vi "OCT.vi"() -> ()   [LabVIEW 2014]
doc: "I. Description:\nThis example demonstrates how to acquire a continuous amount of data (Waveform) using the DAQ device's internal clock.\n\nII. Instructions for Running:\n1. Create an analog input voltage channel.\n2. Set the rate for the sample clock. Additionally, define the sample mode to be continuous.\n3. Call the Start VI to start the acquisition.\n4. Read the waveform data in a loop until the user hits the stop button or an error occurs.\nNote: This example reads data from one or more channels and returns an array of data. Use the Index Array function to access an individual channel of data.\n5. Call the Clear Task VI to clear the Task.\n6. Use the popup dialog box to display an error if any.\n\nIV. I/O Connections Overview:\nMake sure your signal input terminal matches the Physical Channel I/O Control. For further connection information, refer to your hardware reference manual."
uses:
  ATS-VI/ATS_ctl/Device_Ctrl.ctl
  ATS-VI/ATS_ctl/ATS_Async_Ctrl.ctl
  ATS-VI/ATS_ctl/ATS_Async_Mode.ctl
  ATS-VI/ATS_ctl/ATS_DMA_Channel.ctl
  ATS-VI/ATS_ctl/ATS_ReadSamples.ctl
  ATS-VI/ATS_ctl/ATS_Check_Ctrl.ctl
  ATS-VI/ATS_ctl/ClockSource.ctl
  Galvo VIs/galvo_states.ctl
  Signal Processing/processing_states.ctl
  En Face/En Face States.ctl
  Saving Data/Saving Data States.ctl
  Type Defs/OCT Hardware States.ctl
  ATS-VI/ATS_ctl/Range.ctl
  ATS-VI/ATS_ctl/Impedance.ctl
  Type Defs/OCT Imaging Parameters Cluster.ctl
  Signal Processing/Display Raw Data states.ctl
  ATS-VI/ATS_ctl/Record.ctl
  ATS-VI/ATS_ctl/ClockRate.ctl
  ATS-VI/ATS_ctl/ClockEdge.ctl
  ATS-VI/ATS_ctl/Clock.ctl
  ATS-VI/ATS_ctl/Coupling.ctl
  ATS-VI/ATS_ctl/Bandwidth.ctl
  ATS-VI/ATS_ctl/InputCtrl.ctl
  ATS-VI/ATS_ctl/TriggerOperation.ctl
  ATS-VI/ATS_ctl/TriggerEngine.ctl
  ATS-VI/ATS_ctl/ExtTrigRange.ctl
  ATS-VI/ATS_ctl/ExtTrigger.ctl
  ATS-VI/ATS_ctl/Trigger.ctl
  ATS-VI/ATS_ctl/ATS_Global.ctl
  En Face/En Face Depth Parameters.ctl
  DAQ Status States.ctl
  Classes/DAQ/ATS9462/ATS9462 Class.lvclass
  Type Defs/Display States.ctl
  ATS-VI/ATS_ctl/ATS_Async_Setting.ctl
  Type Defs/OCT DAQ Channel Data Type.ctl
panel:
  out "Background Array":u16[](array[numeric])
  in  "Calibrate":bool
  in  "Save Sweep Button":bool
  in  "Linear?":bool
  in  "Data Format":T1
  out "BScan":sgl[][](graph)
  in  "Display":T2
  in  "Save Sweep":bool
  in  "Stop Button":bool
  out "B-Scans Per Buffer":i32=1
  out "Current State":T3=enum."Aquire and Save"
  in  "Channels":tag="Dev2/ao0:1"
  in  "Trigger Source":tag="/Dev2/PFI7"
  in  "Imaging Parameters":T4={"Points Per A-Scan"=0, "A-Scans per B-Scan"=0, "Voltage Range"=1.0, "Card Resolution (bits)"=12}
  out "First Time?":bool=TRUE
  out "Save Data":bool
  in  "Async_Setting":T5
  out "Processing Finished":bool
  in  "OCT Hardware States":T6=enum."Acquire Clock"
  out "Save State":T7=enum."Do Nothing"
  out "Clock Length":u32=9184
  out "Reset DAQ":bool
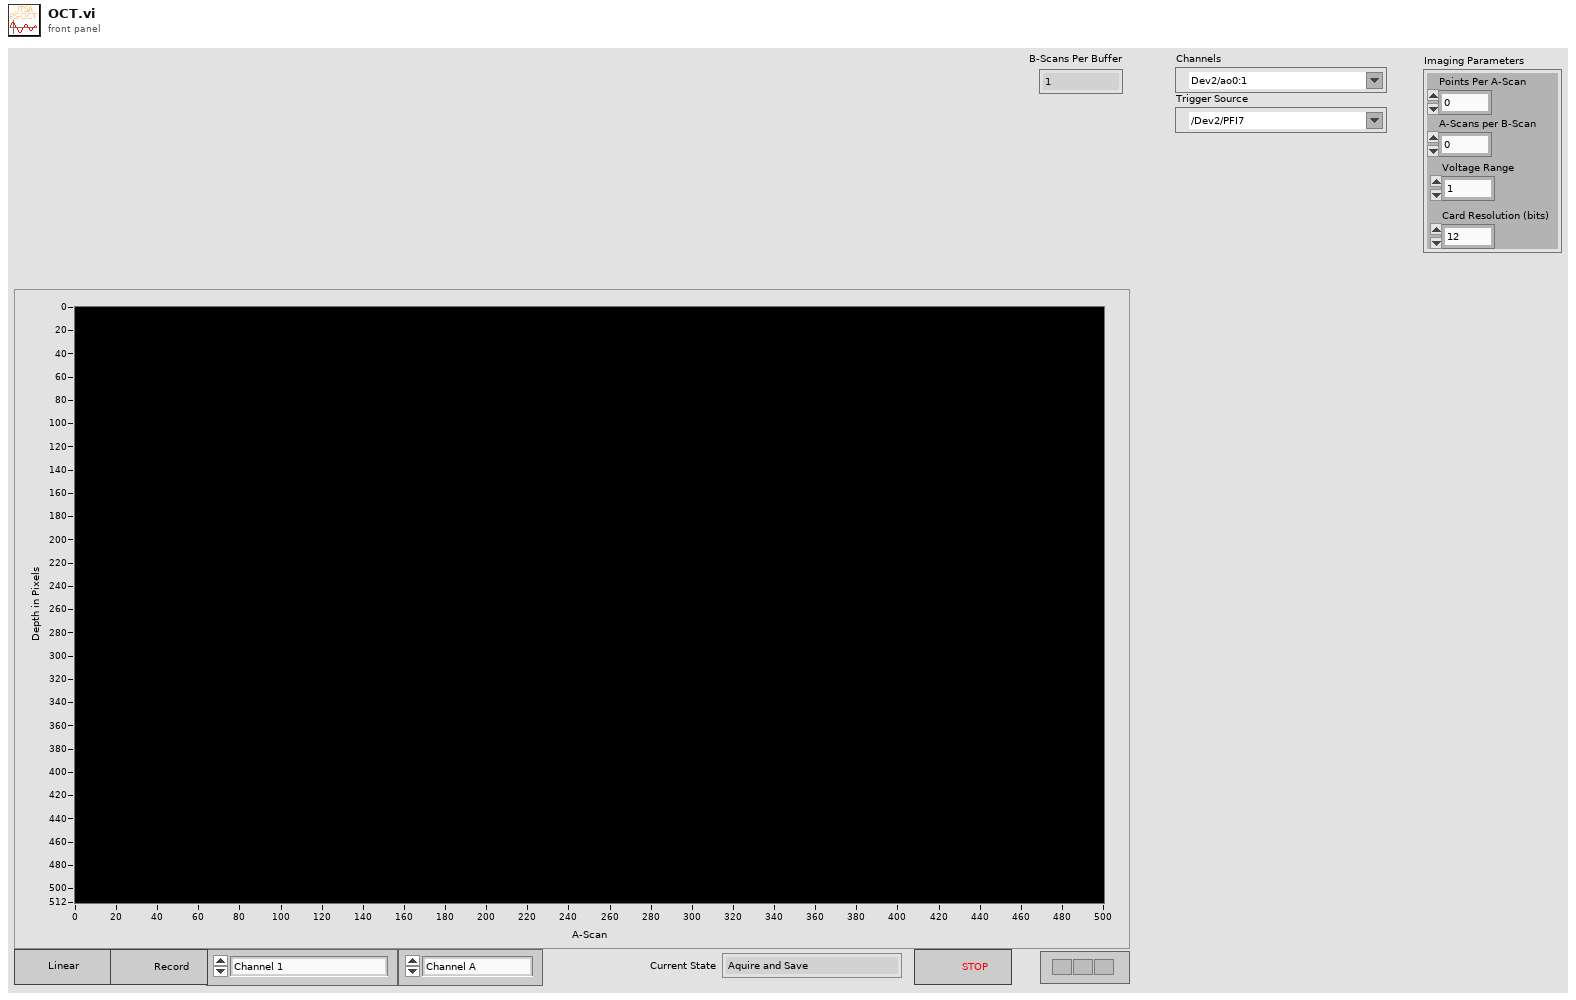
[diagram p1: front panel]
types:
  T1 = typedef "OCT DAQ Channel Data Type.ctl" = enum16{"Channel 1", "Channel 2", "Channel 1 and 2"}
  T2 = typedef "Display States.ctl" = enum16{"Channel A", "Channel B"}
  T3 = typedef "OCT Hardware States.ctl" = enum16{"Acquire Data", "Aquire and Save", "Reset DAQ", "Background Subtraction", "Acquire Background", "Update DAQ Parameters", "Stop", "Set Clock", "Initialize DAQ", "Set Resampling Array"}
  T4 = typedef "OCT Imaging Parameters Cluster.ctl" = cluster{"Points Per A-Scan":i32, "A-Scans per B-Scan":i32, "Voltage Range":sgl, "Card Resolution (bits)":u16}
  T5 = typedef "ATS_Async_Setting.ctl" = cluster{"UseHeader":u32, "Rec/Buffer":u32, "Total_Rec":u32, "DataBuffer":bool, "GetProcessedData":bool}
  T6 = typedef "OCT Hardware States.ctl" = enum16{"Acquire Data", "Aquire and Save", "Allocate OpenCL Memory", "Delete OpenCL Memory", "Background Subtraction", "Acquire Background", "K-Space Calibration", "Update DAQ Parameters", "Initialize Clock", "Stop", "Wait", "Acquire Clock", "Initialize DAQ", "Set Resampling Array"}
  T7 = typedef "Saving Data States.ctl" = enum16{"Get Queue Size", "Get Queue", "Get Timeout", "Flush Queue", "Close Files", "Create Files", "Do Nothing", "Initialize", "Enqueue Data", "Save Data", "Shutdown"}
  T8 = typedef "ATS_Global.ctl" = cluster{"Record":T9, "Clock":T10, "Input A":T14, "Input B":T14, "Trigger":T19}
  T9 = typedef "Record.ctl" = cluster{"Count":u32, "Presize":u32, "Length":u32}
  T10 = typedef "Clock.ctl" = cluster{"ClckSource":T11, "ClckRate":T12, "ClckEdge":T13, "Decimation":u32}
  T11 = typedef "ClockSource.ctl" = enum16{"Internal", "External", "Medium Ext.", "Slow Ext.", "Ext. AC", "Ext. DC", "Ext. (PLL)"}
  T12 = typedef "ClockRate.ctl" = u32
  T13 = typedef "ClockEdge.ctl" = u16
  T14 = typedef "InputCtrl.ctl" = cluster{"Coupling":T15, "Range":T16, "Impedance":T17, "Bandwidth":T18}
  T15 = typedef "Coupling.ctl" = enum16{"AC", "DC"}
  T16 = typedef "Range.ctl" = u32
  T17 = typedef "Impedance.ctl" = enum16{"1M ohms", "50 ohms"}
  T18 = typedef "Bandwidth.ctl" = enum16{"Full Bandwidth", "Reduce Bandwidth"}
  T19 = typedef "Trigger.ctl" = cluster{"TrigOperation":T20, "Timeout (s)":dbl, "Trig. Delay":u32, "Engine X":T21, "Engine Y":T21, "ExtTrigControl":T22}
  T20 = typedef "TriggerOperation.ctl" = enum16{"Only X", "Only Y", "X or Y", "X and Y", "X xor Y", "X and not Y", "not X and Y"}
  T21 = typedef "TriggerEngine.ctl" = cluster{"Source":enum32{"Chan_A", "Chan_B", "External", "Disable"}, "Slope":enum32{"Positive", "Negative"}, "Level":u32}
  T22 = typedef "ExtTrigger.ctl" = cluster{"Coupling":T15, "Range":T23}
  T23 = typedef "ExtTrigRange.ctl" = enum16{"1 V", "5 V", "TTL"}
  T24 = typedef "galvo_states.ctl" = enum16{"Reset", "Reset Galvos?", "Center Galvos", "Register Callback", "Get Scan Parameters", "Show", "Initialize", "Run Raster", "Load Raster", "Run Circle", "Shutdown"}
  T25 = typedef "OCT Hardware States.ctl" = enum16{"Acquire Data", "Initialize Laser", "Initialize Galvos", "Startup", "Reset DAQ", "Background Subtraction", "Acquire Background", "Update DAQ Parameters", "Stop", "Set Clock", "Initialize DAQ", "Set Resampling Array", "Save Sweep", "Configure Laser"}
  T26 = typedef "En Face Depth Parameters.ctl" = cluster{"En Face Start\nDepth":i32, "En Face End\nDepth":i32}
  T27 = typedef "processing_states.ctl" = enum16{"Initialize", "Set Background", "Update Imaging Parameters", "Get Queue", "Process Data", "Get Size", "Flush Data", "Set Reample Array", "Get Last Processed BScan", "Shutdown"}
  T28 = typedef "En Face States.ctl" = enum16{"Save BMP", "Show", "Clear En Face", "Update EnFace"}
  T29 = typedef "Galvo.lvclass/Scanning Cluster.ctl" = cluster{"Fast Axis Offset":sgl, "Slow Axis Offset":sgl, "Slow Axis Amp":sgl, "Fast Axis Amp":sgl, "Scan Pattern":enum16{"Raster"}}
  T30 = typedef "Processed OCT Data.ctl" = cluster{"Intensity A":sgl[][][], "Intensity B":sgl[][][]}
  T31 = typedef "ATS_Async_Ctrl.ctl" = enum16{"SetupDMA", "StartCapture", "Get", "Get_Stream", "Abort", "Stop"}
  T32 = typedef "ATS_ReadSamples.ctl" = cluster{"Offset":i32, "Length":u32}
  T33 = typedef "ATS_DMA_Channel.ctl" = enum16{"Channel_A", "Channel_B", "A & B"}
  T34 = typedef "ATS_Async_Mode.ctl" = enum16{"Continuous", "Triggered", "No-Pre-Trigger", "Traditional"}
  T35 = typedef "ATS_Check_Ctrl.ctl" = enum16{"None", "NO_ATS9462", "ATS9462_Traditional", "Verify Board", "OnBoard Memory", "Board & Memory", "Master/Slave", "NO Master/Slave"}
  T36 = typedef "Device_Ctrl.ctl" = enum16{"Status", "About", "Arm", "ForceTrig", "Abort", "Initialize", "Init (NoPreset)", "Info", "Close", "Calibrate", "SetManually", "LED_ON", "LED_OFF"}
  T37 = typedef "DAQ Status States.ctl" = enum16{"Get", "Show"}
  T38 = typedef "ATS_Async_Status.ctl" = cluster{"Start DMA":bool, "StartCapture":bool, "Valid":bool, "Completed":bool, "InProgress":bool, "Timeout":bool, "Overflow":bool, "Error":bool}
  T39 = typedef "Display Raw Data states.ctl" = enum16{"Add Raw", "Add Processed", "Show"}
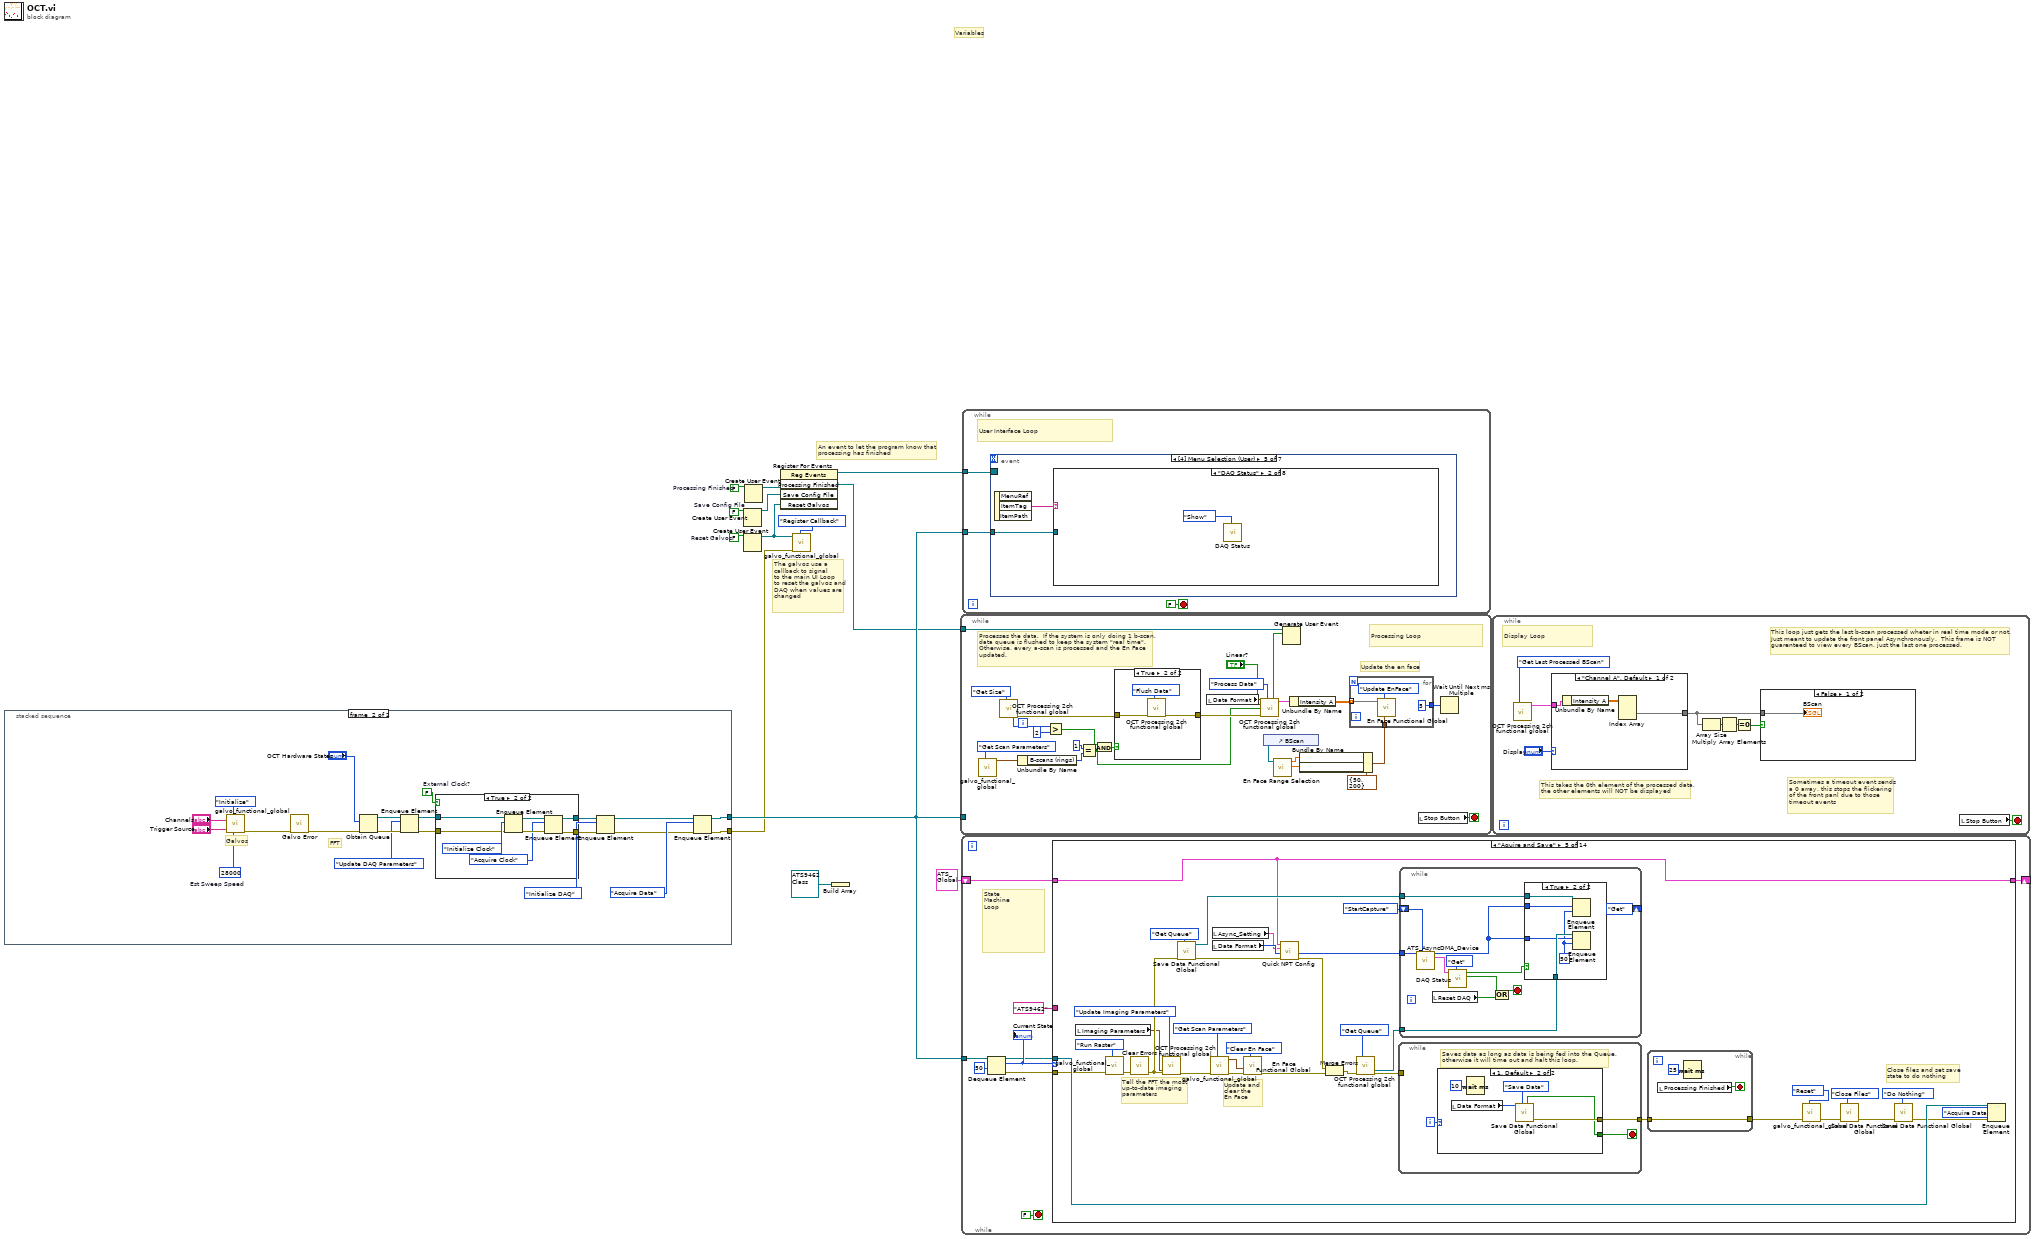
[diagram p0: block diagram]
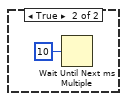
[diagram p3: hidden frame]
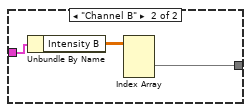
[diagram p4: hidden frame]
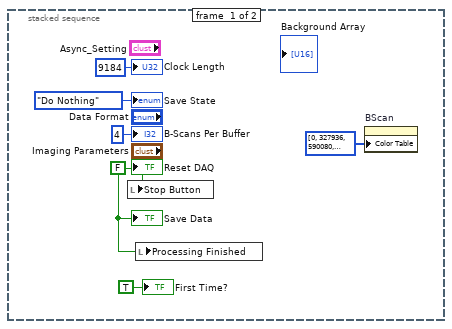
[diagram p5: hidden frame]
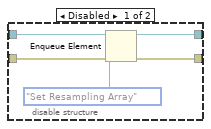
[diagram p7: hidden frame]
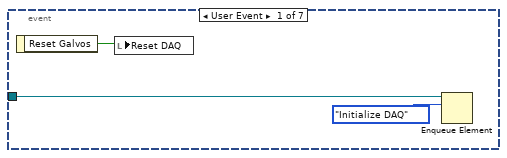
[diagram p8: hidden frame]
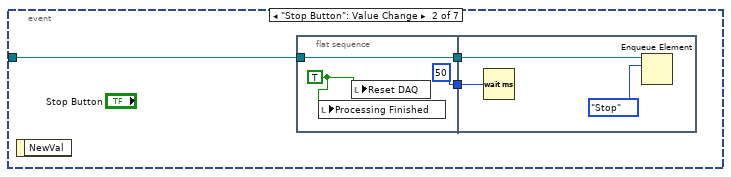
[diagram p9: hidden frame]
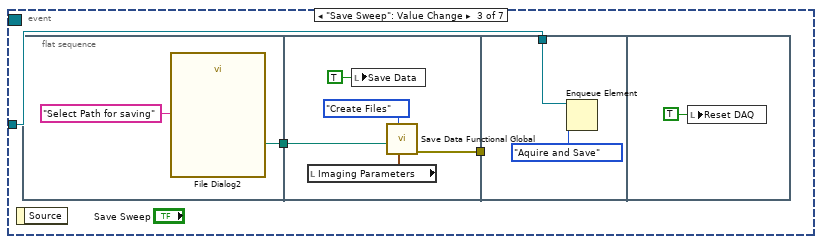
[diagram p10: hidden frame]
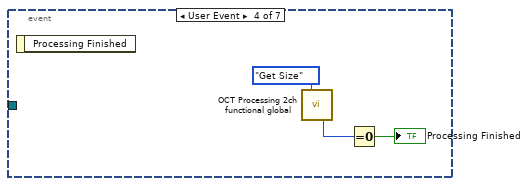
[diagram p11: hidden frame]
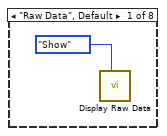
[diagram p12: hidden frame]
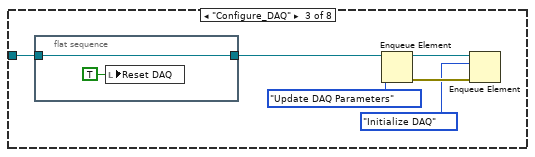
[diagram p13: hidden frame]
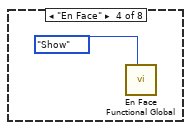
[diagram p14: hidden frame]
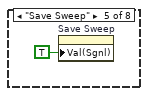
[diagram p15: hidden frame]
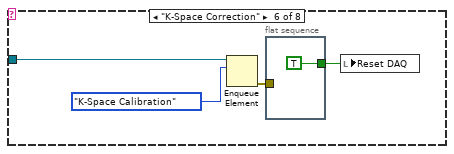
[diagram p16: hidden frame]
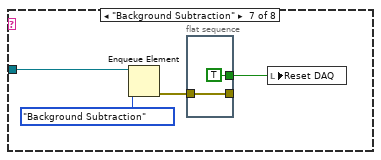
[diagram p17: hidden frame]
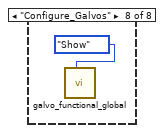
[diagram p18: hidden frame]
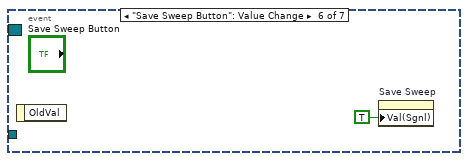
[diagram p19: hidden frame]
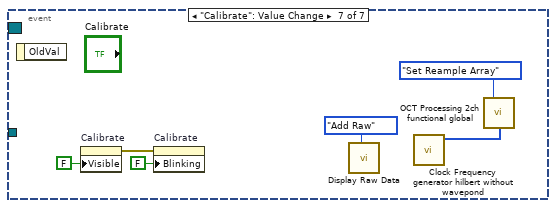
[diagram p20: hidden frame]
diagram:
  w7 = FALSE  # Reset Galvos
  w10 = FALSE  # Save Config File
  w13 = FALSE  # Processing Finished
  # "The galvos use a \ncallback to signal\nto the main UI Loop\nto reset the galvos and\nDAQ when values are\nchanged"
  # "An event to let the program know that\nprocessing has finished"
  # "Variables"
  n1 = stacked-sequence {
    tunnel: [_ w28] -> w11
    tunnel: [_ w27] -> w3
    frame #0 {
      w16 = FALSE ("Sweep Ready for saving")
      n2 = local write "Stop Button"(w16) -> ()
      n3 = local write "Processing Finished"(w16) -> ()
      n4 = property on="BScan" class="IntGraph (strict)"("Color Table"=u32[] [0, 327936, 590080, 852224, 983296, 1114624, 1180160, 1311232, 1442304, 1573632, 1704704, 1770240, 1901312, 1966848, 2098176, 2163712, 2294784, 2491392, 2557184, 2688256, 2753792, 2884864, 2950656, 3081728, 3147264, 3344129, 3475457, 3540993, 3672321, 3738113, 3869185, 3934977, 4066305, 4197633, 4328961, 4394497, 4460289, 4591617, 4657409, 4788481, 4854273, 4985601, 5116929, 5248257, 5314049, 5379841, 5511169, 5576961, 5708033, 5773825, 5905153, 6036482, 6167810, 6233346, 6299138, 6430466, 6496258, 6562050, 6693634, 6759426, 6890754, 7022082, 7087874, 7153666, 7284994, 7350786, 7482114, 7547906, 7613698, 7745026, 7876354, 8007682, 8073474, 8139522, 8205314, 8336642, 8467970, 8533763, 8599555, 8665347, 8731139, 8862467, 8993795, 9059587, 9125380, 9191428, 9257220, 9388548, 9454340, 9520132, 9585924, 9717253, 9848837, 9914629, 9980165, 10045957, 10177541, 10243334, 10309126, 10375174, 10440966, 10572294, 10703623, 10769416, 10835208, 10901256, 10967049, 11033097, 11033609, 11099401, 11165450, 11231242, 11231754, 11297547, 11363339, 11429131, 11495180, 11495692, 11561740, 11693069, 11758861, 11759373, 11825165, 11891214, 11957006, 12022799, 12023311, 12089103, 12220944, 12286736, 12286736, 12352529, 12418577, 12484370, 12550162, 12615954, 12681747, 12747796, 12813588, 12813845, 12879894, 12945686, 13077015, 13142808, 13143064, 13208856, 13274905, 13340697, 13340953, 13472282, 13538075, 13604379, 13670172, 13735964, 13801757, 13867550, 13933343, 13999392, 13999648, 14065441, 14131234, 14197027, 14197541, 14263334, 14329383, 14395176, 14460969, 14592553, 14658346, 14724139, 14789932, 14790189, 14856238, 14922287, 14988080, 15053873, 15054130, 15119923, 15185972, 15251765, 15317559, 15383353, 15449146, 15449660, 15515454, 15515968, 15516226, 15582021, 15582278, 15582536, 15648587, 15648844, 15714639, 15714897, 15715155, 15780949, 15781463, 15847256, 15847770, 15848028, 15913823, 15914081, 15979875, 15980133, 15980391, 16046441, 16046444, 16046703, 16046705, 16112500, 16113015, 16113274, 16113277, 16179072, 16179330, 16179588, 16245384, 16245387, 16245389, 16245648, 16311443, 16376982, 16377241, 16377499, 16443294, 16443553, 16443555, 16443815, 16509866, 16510124, 16510127, 16575923, 16575924, 16576182, 16576441, 16576443, 16576702, 16576705, 16576963, 16577222, 16577224, 16577482, 16577485, 16577743, 16577745, 16578004, 16578262, 16578264, 16578523, 16578782, 16579040, 16579299, 16579301, 16579303, 16579562, 16579821]) -> ()  [unwired: 2 in, 2 out]
      "B-Scans Per Buffer" <- 4 ("B-Scans Per Buffer")
      "Clock Length" <- u32 9184 ("Clock Length")
      "Save State" <- Saving_Data_States."Do Nothing" ("Save State")
      "Reset DAQ" <- w16
      "Save Data" <- w16
      "First Time?" <- TRUE ("First Time?")
    }
    frame #1 {
      w32 = 28000  # Est Sweep Speed
      w33 = FALSE  # External Clock?
      # "FFT"
      # "Galvos"
      n5 = call "galvo_functional_global.vi"("Est Sweep Speed"=w32, "State"=galvo_states."Initialize", "Trigger Source"="Trigger Source", "Analog Output"="Channels") -> ("error out"=w21:errorcluster)  [unwired: 6 in, 1 out]
      n6 = call "Galvo Error.vi"("error in (no error)"=w21) -> ("error out"=w20:errorcluster)  [unwired: 10 in]
      n7 = Obtain Queue(element data type="OCT Hardware States", error in (no error)=w20) -> (queue out=w30:refnum<queue>, error out=w31:errorcluster)  [unwired: 3 in, 1 out]
      n8 = Enqueue Element(queue=w30, element=OCT_Hardware_States."Update DAQ Parameters", error in (no error)=w31) -> (queue out=w25:refnum<queue>, error out=w24:errorcluster)  [unwired: 1 in, 1 out]
      n9 = case shown="True" w33 {
        tunnel: [w41 w57] -> w40
        tunnel: [w42 w56] -> w39
        tunnel: w25 -> [w44 w53]
        tunnel: w24 -> [w43 w52]
        frame False {
          n10 = disable-structure shown="Enabled" {
            disable-tunnel: w44 -> [w49 w51]
            disable-tunnel: w43 -> [w48 w50]
            disable-tunnel: [w47 w50] -> w42
            disable-tunnel: [w46 w51] -> w41
            frame Disabled {
              n11 = Enqueue Element(queue=w49, element=OCT_Hardware_States."Set Resampling Array", error in (no error)=w48) -> (queue out=w46:refnum<queue>, error out=w47:errorcluster)  [unwired: 1 in, 1 out]
            }
            frame Enabled {
            }
          }
        }
        frame True {
          n12 = Enqueue Element(queue=w53, element=OCT_Hardware_States."Initialize Clock", error in (no error)=w52) -> (queue out=w59:refnum<queue>, error out=w58:errorcluster)  [unwired: 1 in, 1 out]
          n13 = Enqueue Element(queue=w59, element=OCT_Hardware_States."Acquire Clock", error in (no error)=w58) -> (queue out=w57:refnum<queue>, error out=w56:errorcluster)  [unwired: 1 in, 1 out]
        }
      }
      n14 = Enqueue Element(queue=w40, element=OCT_Hardware_States."Initialize DAQ", error in (no error)=w39) -> (queue out=w22:refnum<queue>, error out=w23:errorcluster)  [unwired: 1 in, 1 out]
      n15 = Enqueue Element(queue=w22, element=OCT_Hardware_States."Acquire Data", error in (no error)=w23) -> (queue out=w28:refnum<queue>, error out=w27:errorcluster)  [unwired: 1 in, 1 out]
    }
  }
  n16 = Create User Event(user event datatype=w10) -> (user event=w9:refnum<user-event>)  [unwired: 1 in, 1 out]
  n17 = Create User Event(user event datatype=w7) -> (user event=w6:refnum<user-event>)  [unwired: 1 in, 1 out]
  n18 = Create User Event(user event datatype=w13) -> (user event=w8:refnum<user-event>)  [unwired: 1 in, 1 out]
  n19 = register-events(w8, w9, w6) -> (reference out=w12:refnum<event-registration>)  [unwired: 2 in, 1 out]
  n20 = call "galvo_functional_global.vi"("State"=galvo_states."Register Callback", "error in (no error)"=w3, "user event out"=w6) -> ()  [unwired: 7 in, 2 out]
  n21 = Build Array(refnum<class "ATS9462 Class.lvclass"> refnum ("ATS9462 Class.lvclass")) -> (w1:refnum<class "ATS9462 Class.lvclass">[])
  n22 = while {
    tunnel: w8 -> [w75]
    tunnel: w11 -> [_]
    stop <- w85 stop-if-true
    # "Processing Loop"
    # "Update the en face"
    # "Processes the data.  If the system is only doing 1 b-scan, \ndata queue is flushed to keep the system \"real time\".\nOtherwise, every a-scan is processed and the En Face\nupdated."
    n23 = call "galvo_functional_global.vi"("State"=galvo_states."Get Scan Parameters") -> ("Scanning Output"=w69:T29)  [unwired: 9 in, 1 out]
    n24 = call "OCT Processing 2ch functional global.vi"("State"=processing_states."Get Size") -> ("# elements in queue"=w81:i32, "error out"=w72:errorcluster)  [unwired: 10 in, 3 out]
    n25 = Unbundle By Name(w69) -> ("B-scans (rings)"=w77:u32)
    n26 = Greater?(x=w81, y=2) -> (0:w82:bool)
    n27 = Equal?(x=u32 1, y=w77) -> (x = y?=w65:bool)
    n28 = And(x=w82, y=w65) -> (x .and. y?=w70:bool)
    n29 = case shown="True" w70 {
      tunnel: w72 -> [w90 w93]
      tunnel: [w90 w92] -> w71
      frame False {
      }
      frame True {
        n30 = call "OCT Processing 2ch functional global.vi"("State"=processing_states."Flush Data", "error in (no error)"=w93) -> ("error out"=w92:errorcluster)  [unwired: 9 in, 4 out]
      }
    }
    n31 = local read "Data Format"() -> (w76:T1)
    n32 = call "OCT Processing 2ch functional global.vi"("Data Format"=w76, "State"=processing_states."Process Data", "Linear?"="Linear?", "Real Time"=w65, "error in (no error)"=w71) -> ("Time Out"=w74:bool, "Processed OCT Data"=w79:T30)  [unwired: 6 in, 3 out]
    n33 = control-ref of="BScan"() -> (w64:refnum<vi>)
    n34 = call "En Face Range Selection.vi"("IntensityGraph in"=w64) -> ("Lower En Face"=w61:dbl, "Upper En Face"=w62:dbl)  [unwired: 9 in]
    n35 = Generate User Event(user event=w75, event data cluster=w74) -> ()  [unwired: 2 in, 2 out]
    n36 = Unbundle By Name(w79) -> ("Intensity A"=w73:sgl[][][])
    n37 = Bundle By Name(cluster=T26 {"En Face Start\nDepth"=50, "En Face End\nDepth"=200} ("En Face Parameters"), "En Face Start\nDepth"=w62, "En Face End\nDepth"=w61) -> (w60:T26)
    n38 = for {
      tunnel: w73 -> [w88] mode=indexing
      tunnel: [u32 5 ("millisecond multiple")] -> w67
      tunnel: w60 -> [w86]
      n39 = call "En Face Functional Global.vi"(6:w86, 7:En_Face_States."Update EnFace" ("En Face States"), "Intensity Graph 2"=w88) -> ()  [unwired: 7 in, 2 out]
    }
    n40 = local read "Stop Button"() -> (w85:bool)
    n41 = Wait Until Next ms Multiple(millisecond multiple=w67) -> ()  [unwired: 1 out]
  }
  n42 = while {
    tunnel: w11 -> [w102]
    shift-right: [w96] -> _
    shift-left: T8 {"Record"={"Count"=0, "Presize"=0, "Length"=0}, "Clock"={"ClckSource"=enum."Internal", "ClckRate"=0, "ClckEdge"=0, "Decimation"=0}, "Input A"={"Coupling"=enum."DC", "Range"=12, "Impedance"=enum."1M ohms", "Bandwidth"=enum."Full Bandwidth"}, "Input B"={"Coupling"=enum."DC", "Range"=12, "Impedance"=enum."1M ohms", "Bandwidth"=enum."Full Bandwidth"}, "Trigger"={"TrigOperation"=enum."Only X", "Timeout (s)"=-1.0, "Trig. Delay"=0, "Engine X"={"Source"=enum."Chan_A", "Slope"=enum."Positive", "Level"=0}, "Engine Y"={"Source"=enum."Chan_A", "Slope"=enum."Positive", "Level"=0}, "ExtTrigControl"={"Coupling"=enum."AC", "Range"=enum."1 V"}}} ("Value") -> [w95]
    stop <- FALSE stop-if-true
    # "State\nMachine\nLoop"
    n43 = Dequeue Element(queue=w102, timeout in ms (-1)=50) -> (queue out=w98:refnum<queue>, element=w100:T6, error out=w99:errorcluster)  [unwired: 1 in, 1 out]
    "Current State" <- w100
    n44 = case shown="\"Aquire and Save\"" w100 {
      tunnel: w99 -> [_ w146 w203 w255 w309 _ w367 _ _ _ w405 w413 _ _]
      tunnel: w98 -> [_ _ w204 w254 w323 _ w368 _ _ _ w406 w411 _ _]
      tunnel: "ATS9462" ("BoardToVerify") -> [_ w160 _ _ _ _ _ w375 _ _ _ _ _ _]
      tunnel: [w119 w154 w220 w266 w298 w357 w359 w374 w390 w391 w401 w415 w418 w419] -> w96
      tunnel: w95 -> [w119 w153 w220 w266 w298 w357 w359 w374 w390 _ w401 w415 w418 w419]
      frame "Acquire Clock" {
        w106 = 0 ("DeviceIn")
        n45 = local read "Clock Length"() -> (w108:u32)
        n46 = local read "Async_Setting"() -> (w104:T5)
        n47 = Bundle By Name(cluster=w104, "UseHeader"=u32 0, "Rec/Buffer"=u32 125, "Total_Rec"=u32 0) -> (w105:T5)
        n48 = Unbundle By Name(w119) -> ("Record.Presize"=w109:u32)
        n49 = Bundle By Name(cluster=T32 {"Offset"=0, "Length"=0} ("ReadSamples"), "Length"=w108, "Offset"=w109) -> (w107:T32)
        n50 = call "ATS_AsyncDMA_Device.vi"("DeviceIn"=w106, "ATS_Async_Ctrl"=ATS_Async_Ctrl."SetupDMA" ("ATS_DMA_Ctrl"), "Async_Mode"=ATS_Async_Mode."Traditional", "Async_Setting"=w105, "Channel"=ATS_DMA_Channel."Channel_B", "ReadSamples"=w107, "Start Now / Wait"=TRUE) -> ("Buffer"=w114:u16[])  [unwired: 4 in, 4 out]
        n51 = while {
          tunnel: w114 -> [_]
          shift-right: [ATS_Async_Ctrl."Get" ("ATS_Async_Ctrl")] -> _
          shift-left: ATS_Async_Ctrl."StartCapture" ("ATS_Async_Ctrl") -> [w128]
          tunnel: w106 -> [w123]
          stop <- w126 stop-if-true
          n52 = call "ATS_AsyncDMA_Device.vi"("DeviceIn"=w123, "ATS_Async_Ctrl"=w128) -> ("Buffer"=w121:u16[], "Async_Status"=w120:T38)  [unwired: 9 in, 3 out]
          n53 = Unbundle By Name(w120) -> ("Valid"=w122:bool, "Completed"=w130:bool, "Start DMA"=w131:bool, "Timeout"=w132:bool, "Error"=w129:bool)
          n54 = local read "Clock Length"() -> (w124:u32)
          n55 = Compound Arithmetic op=OR(w130, invert w131, w132, w129) -> (w125:bool)
          n56 = case shown="True" w122 {
            selector: w122 -> [w133 w136]
            tunnel: w121 -> [_ w135]
            tunnel: [w133 w136] -> w126
            tunnel: w125 -> [_ _]
            tunnel: w124 -> [_ w134]
            frame False {
            }
            frame True {
              n57 = Array Subset(array=w135, length=w134) -> (w137:u16[])  [unwired: 1 in]
              n58 = call "Clock Frequency generator hilbert.vi"(7:6300.0 ("Sweep Speed"), "Acquisition speed (S/s)"=180000000.0 ("Sweep Speed"), "k-space signal in"=w137, "number of frequency updates"=4385) -> ("Error Out"=w142:errorcluster, "frequency\nsteps"=w141:i32)  [unwired: 6 in]
              n59 = call "wavepond sequence.vi"("Error In"=w142, "Number of updates"=w141) -> ()  [unwired: 9 in, 1 out]
            }
          }
        }
      }
      frame "Initialize DAQ" {
        # "B-Scans per buffer should be around 4 if \ntaking more than 1 to minimize data transfer"
        # "If B Scans is 1, set total records to 0,\notherwise it should be A-Scans Per\nBScan times BScans"
        # "BScans Per Buffer"
        n60 = local read "First Time?"() -> (w157:bool)
        n61 = case shown="False" w157 {
          tunnel: [w186 w196] -> w182
          tunnel: w160 -> [_ w192]
          tunnel: [FALSE ("First Time?") FALSE ("First Time?")] -> w156
          frame False {
            n62 = flat-sequence {
              tunnel: [w188] -> w186
              frame #0 {
                w188 = 0 ("DeviceIn")
                n63 = call "ATS_AsyncDMA_Device.vi"("DeviceIn"=w188, "ATS_Async_Ctrl"=ATS_Async_Ctrl."Stop") -> ("ReadSamples_Out"=w191:T32)  [unwired: 9 in, 4 out]
                n64 = call "ATS_AsyncDMA_Device.vi"("DeviceIn"=w188, "ATS_Async_Ctrl"=ATS_Async_Ctrl."Abort", "ReadSamples"=w191) -> ()  [unwired: 8 in, 5 out]
              }
            }
          }
          frame True {
            n65 = call "ATS_Device.vi"("BoardToVerify"=w192, "ATS_Check"=ATS_Check_Ctrl."Verify Board", "DevCtrl"=Device_Ctrl."Initialize", "DeviceIn"=0 ("Device")) -> ("error out"=w194:errorcluster, "DeviceOut"=w198:i32)  [unwired: 1 in, 5 out]
            n66 = call "ATS_Device.vi"("error in (no error)"=w194, "DevCtrl"=Device_Ctrl."Abort", "DeviceIn"=w198) -> ("DeviceOut"=w196:i32)  [unwired: 2 in, 6 out]
          }
        }
        n67 = flat-sequence {
          tunnel: w146 -> [w184]
          tunnel: [w184] -> w147
          frame #0 {
            n68 = local write "Processing Finished"(FALSE ("Reset DAQ")) -> ()
            n69 = local write "Reset DAQ"(FALSE ("Reset DAQ")) -> ()
          }
        }
        n70 = call "Save Data Functional Global.vi"("States"=Saving_Data_States."Flush Queue", "error in (no error)"=w147) -> ("error out"=w149:errorcluster)  [unwired: 6 in, 3 out]
        n71 = call "OCT Processing 2ch functional global.vi"("State"=processing_states."Flush Data", "error in (no error)"=w149) -> ("error out"=w145:errorcluster)  [unwired: 9 in, 4 out]
        n72 = local write "First Time?"(w156) -> ()
        n73 = Unbundle By Name(w153) -> ("Record.Length"=w161:u32)
        n74 = call "ATS_MS_Set_Device.vi"("Set_Manually (F)"=FALSE, "Setup_In"=w153, "DeviceIn"=w182) -> ("Setup_Out"=w154:T8)  [unwired: 3 in, 5 out]
        n75 = call "galvo_functional_global.vi"("State"=galvo_states."Get Scan Parameters", "error in (no error)"=w145) -> ("Scanning Output"=w152:T29)  [unwired: 8 in, 1 out]
        n76 = Unbundle By Name(w152) -> ("B-scans (rings)"=w167:u32, "A(cluster)/B"=w177:u32, "B-scans (rings)"=w172:u32, "A(cluster)/B"=w171:u32, "B-scans (rings)"=w169:u32, "A(cluster)/B"=w163:u32)
        n77 = local read "Async_Setting"() -> (w159:T5)
        n78 = Not Equal?(x=w169, y=u32 1 ("x")) -> (x != y?=w170:bool)
        n79 = Equal?(x=u32 1, y=w167) -> (x = y?=w173:bool)
        n80 = local read "B-Scans Per Buffer"() -> (w155:i32)
        n81 = Select(t=u32 4 ("y"), s=w173, f=w155) -> (s? t:f=w175:u32)
        n82 = Multiply(x=w172, y=w171) -> (x*y=w166:u32)
        n83 = Select(t=w166, s=w170, f=u32 0 ("Total_Rec")) -> (s? t:f=w180:u32)
        n84 = Multiply(x=w175, y=w177) -> (x*y=w178:u32)
        n85 = Bundle By Name(cluster=T4 {"Points Per A-Scan"=0, "A-Scans per B-Scan"=0, "Voltage Range"=4.0, "Card Resolution (bits)"=16} ("Imaging Parameters"), "Points Per A-Scan"=w161, "A-Scans per B-Scan"=w163, "Voltage Range"=sgl 4.0, "Card Resolution (bits)"=u16 16) -> (w162:T4)
        n86 = Bundle By Name(cluster=w159, "UseHeader"=u32 0, "Rec/Buffer"=w178, "Total_Rec"=w180) -> (w158:T5)
        n87 = local write "Async_Setting"(w158) -> ()
        n88 = local write "Imaging Parameters"(w162) -> ()
      }
      frame "Acquire Data", Default {
        # "Update and \nclear the \nEn Face"
        # "Tell the FFT the most\nup-to-date imaging\nparameters"
        n89 = Enqueue Element(queue=w204, element=OCT_Hardware_States."Initialize DAQ", error in (no error)=w203) -> (error out=w201:errorcluster)  [unwired: 1 in, 2 out]
        n90 = local read "Imaging Parameters"() -> (w225:T4)
        n91 = call "galvo_functional_global.vi"("State"=galvo_states."Run Raster", "error in (no error)"=w201) -> ("error out"=w216:errorcluster)  [unwired: 8 in, 1 out]
        n92 = local read "Async_Setting"() -> (w224:T5)
        n93 = call <vilib>:"Clear Errors.vi"("error in (no error)"=w216) -> ("error out"=w215:errorcluster)  [unwired: 5 in, 1 out]
        n94 = call "OCT Processing 2ch functional global.vi"("State"=processing_states."Update Imaging Parameters", "Input Parameters"=w225, "error in (no error)"=w215) -> ("error out"=w208:errorcluster)  [unwired: 8 in, 4 out]
        n95 = local read "Data Format"() -> (w227:T1)
        n96 = call "galvo_functional_global.vi"("State"=galvo_states."Get Scan Parameters", "error in (no error)"=w208) -> ("error out"=w209:errorcluster, "Scanning Output"=w217:T29)  [unwired: 8 in]
        n97 = call "Quick NPT Config.vi"("error in (no error)"=w201, "Data Format"=w227, "Async_Setting"=w224, "Value"=w220) -> ("error out"=w205:errorcluster, "Device Out"=w230:i32, 3:w210)  [unwired: 4 in]
        n98 = call "En Face Functional Global.vi"(7:En_Face_States."Clear En Face" ("En Face States"), "Error In"=w209, 9:w217) -> ("Error Out"=w207:errorcluster)  [unwired: 7 in, 1 out]
        n99 = Merge Errors(w205, w207) -> (w206:errorcluster)
        n100 = call "OCT Processing 2ch functional global.vi"("State"=processing_states."Get Queue", "error in (no error)"=w206) -> ("queue out"=w222:refnum<queue>, "error out"=w214:errorcluster)  [unwired: 9 in, 3 out]
        n101 = while {
          tunnel: w230 -> [w250]
          shift-right: [ATS_Async_Ctrl."Get" ("ATS_Async_Ctrl")] -> _
          shift-left: ATS_Async_Ctrl."StartCapture" ("ATS_Async_Ctrl") -> [w249]
          tunnel: w222 -> [w245]
          tunnel: [w244] -> w221
          tunnel: w210 -> [w243]
          tunnel: w214 -> [w239]
          tunnel: [w239] -> w213
          stop <- w244 stop-if-true
          n102 = call "ATS_AsyncDMA_Device.vi"("DeviceIn"=w250, "ATS_Async_Ctrl"=w249) -> ("Buffer"=w247:u16[], "Async_Status"=w242:T38)  [unwired: 9 in, 3 out]
          n103 = local read "Reset DAQ"() -> (w246:bool)
          n104 = call "DAQ Status.vi"("Enum"=DAQ_Status_States."Get", "Async_Status"=w242) -> ("DAQ Error?"=w240:bool, "Valid"=w241:bool)  [unwired: 8 in]
          n105 = Compound Arithmetic op=OR(w240, w246) -> (w244:bool)
          n106 = case shown="True" w241 {
            tunnel: w247 -> [_ w251]
            tunnel: w245 -> [_ w253]
            tunnel: w243 -> [_ _]
            frame False {
              # "Do nothing"
            }
            frame True {
              n107 = Enqueue Element(queue=w253, element=w251, timeout in ms (-1)=50) -> ()  [unwired: 1 in, 3 out]
            }
          }
        }
        n108 = while {
          tunnel: w221 -> [w237]
          tunnel: [w234] -> w212
          tunnel: w213 -> [w234]
          stop <- w231 stop-if-true
          n109 = local read "Processing Finished"() -> (w236:bool)
          n110 = Wait (ms)(milliseconds to wait=u32 25) -> ()  [unwired: 1 out]
          n111 = local read "Reset DAQ"() -> (w232:bool)
          n112 = And(x=w237, y=w236) -> (x .and. y?=w233:bool)
          n113 = Or(x=w233, y=w232) -> (x .or. y?=w231:bool)
        }
        n114 = call "galvo_functional_global.vi"("State"=galvo_states."Reset", "error in (no error)"=w212) -> ()  [unwired: 8 in, 2 out]
      }
      frame "Acquire Background" {
        # "Update and \nclear the \nEn Face"
        # "Tell the FFT the most\nup-to-date imaging\nparameters"
        n115 = local read "Imaging Parameters"() -> (w268:T4)
        n116 = call "galvo_functional_global.vi"("State"=galvo_states."Run Raster", "error in (no error)"=w255) -> ("error out"=w263:errorcluster)  [unwired: 8 in, 1 out]
        n117 = local read "Async_Setting"() -> (w267:T5)
        n118 = call <vilib>:"Clear Errors.vi"("error in (no error)"=w263) -> ("error out"=w262:errorcluster)  [unwired: 5 in, 1 out]
        n119 = call "OCT Processing 2ch functional global.vi"("State"=processing_states."Update Imaging Parameters", "Input Parameters"=w268, "error in (no error)"=w262) -> ("error out"=w261:errorcluster)  [unwired: 8 in, 4 out]
        n120 = local read "Data Format"() -> (w269:T1)
        n121 = call "galvo_functional_global.vi"("State"=galvo_states."Get Scan Parameters", "error in (no error)"=w261) -> ("error out"=w259:errorcluster)  [unwired: 8 in, 1 out]
        n122 = call "Quick NPT Config.vi"("error in (no error)"=w255, "Data Format"=w269, "Async_Setting"=w267, "Value"=w266) -> ("error out"=w260:errorcluster, "Device Out"=w272:i32)  [unwired: 5 in]
        n123 = Merge Errors(w260, w259) -> (w256:errorcluster)
        n124 = while {
          tunnel: w272 -> [w282]
          shift-right: [ATS_Async_Ctrl."Get" ("ATS_Async_Ctrl")] -> _
          shift-left: ATS_Async_Ctrl."StartCapture" ("ATS_Async_Ctrl") -> [w281]
          tunnel: w256 -> [w278]
          tunnel: [w278] -> w257
          stop <- w274 stop-if-true
          n125 = local read "Imaging Parameters"() -> (w275:T4)
          n126 = call "ATS_AsyncDMA_Device.vi"("DeviceIn"=w282, "ATS_Async_Ctrl"=w281) -> ("Buffer"=w276:u16[], "Async_Status"=w279:T38)  [unwired: 9 in, 3 out]
          n127 = call "DAQ Status.vi"("Enum"=DAQ_Status_States."Get", "Async_Status"=w279) -> ("Valid"=w277:bool)  [unwired: 8 in, 1 out]
          n128 = case shown="True" w277 {
            selector: w277 -> [_ w287]
            tunnel: w276 -> [_ w291]
            tunnel: w275 -> [_ w290]
            tunnel: [FALSE w287] -> w274
            frame False {
            }
            frame True {
              n129 = Unbundle By Name(w290) -> ("A-Scans per B-Scan"=w289:i32, "Points Per A-Scan"=w288:i32)
              n130 = Reshape Array(w291, w289, w288) -> (w285:u16[][])
              n131 = call "Average BScan.vi"("B-Scan In"=w285) -> ("Averaged BScan"=w284:dbl[])  [unwired: 10 in]
              n132 = call "OCT Processing 2ch functional global.vi"("State"=processing_states."Set Background", "Background"=w284) -> ()  [unwired: 9 in, 5 out]
            }
          }
        }
        n133 = Enqueue Element(queue=w254, element=OCT_Hardware_States."Set Resampling Array", error in (no error)=w257) -> ()  [unwired: 1 in, 3 out]
      }
      frame "Aquire and Save" {
        # "Close files and set save \nstate to do nothing"
        # "Update and \nclear the \nEn Face"
        # "Tell the FFT the most\nup-to-date imaging\nparameters"
        n134 = local read "Imaging Parameters"() -> (w321:T4)
        n135 = call "galvo_functional_global.vi"("State"=galvo_states."Run Raster", "error in (no error)"=w309) -> ("error out"=w306:errorcluster)  [unwired: 8 in, 1 out]
        n136 = call <vilib>:"Clear Errors.vi"("error in (no error)"=w306) -> ("error out"=w326:errorcluster)  [unwired: 5 in, 1 out]
        n137 = call "OCT Processing 2ch functional global.vi"("State"=processing_states."Update Imaging Parameters", "Input Parameters"=w321, "error in (no error)"=w326) -> ("error out"=w295:errorcluster)  [unwired: 8 in, 4 out]
        n138 = call "Save Data Functional Global.vi"("States"=Saving_Data_States."Get Queue", "error in (no error)"=w326) -> ("error out"=w297:errorcluster, "Saving Queue Out"=w312:refnum<queue>)  [unwired: 6 in, 2 out]
        n139 = call "galvo_functional_global.vi"("State"=galvo_states."Get Scan Parameters", "error in (no error)"=w295) -> ("error out"=w296:errorcluster, "Scanning Output"=w307:T29)  [unwired: 8 in]
        n140 = local read "Async_Setting"() -> (w300:T5)
        n141 = local read "Data Format"() -> (w301:T1)
        n142 = call "En Face Functional Global.vi"(7:En_Face_States."Clear En Face" ("En Face States"), "Error In"=w296, 9:w307) -> ("Error Out"=w294:errorcluster)  [unwired: 7 in, 1 out]
        n143 = call "Quick NPT Config.vi"("error in (no error)"=w297, "Data Format"=w301, "Async_Setting"=w300, "Value"=w298) -> ("error out"=w293:errorcluster, "Device Out"=w299:i32)  [unwired: 5 in]
        n144 = Merge Errors(w293, w294) -> (w292:errorcluster)
        n145 = call "OCT Processing 2ch functional global.vi"("State"=processing_states."Get Queue", "error in (no error)"=w292) -> ("queue out"=w314:refnum<queue>, "error out"=w316:errorcluster)  [unwired: 9 in, 3 out]
        n146 = while {
          tunnel: w316 -> [_]
          tunnel: [w332] -> w303
          i -> [w331]
          stop <- w330 stop-if-true
          # "Saves data as long as data is being fed into the Queue,\notherwise it will time out and halt this loop."
          n147 = case shown="1, Default" w331 {
            tunnel: [FALSE w335] -> w330
            tunnel: [_ w336] -> w332
            frame 0 {
              # "Wait for data to Q up"
              n148 = Wait (ms)(milliseconds to wait=u32 500) -> ()  [unwired: 1 out]
            }
            frame 1, Default {
              n149 = local read "Data Format"() -> (w338:T1)
              n150 = Wait (ms)(milliseconds to wait=u32 10) -> ()  [unwired: 1 out]
              n151 = call "Save Data Functional Global.vi"("States"=Saving_Data_States."Save Data", "Data Format"=w338) -> ("error out"=w336:errorcluster, "Time Out"=w335:bool)  [unwired: 6 in, 2 out]
            }
          }
        }
        n152 = while {
          shift-right: [ATS_Async_Ctrl."Get" ("ATS_Async_Ctrl")] -> _
          shift-left: ATS_Async_Ctrl."StartCapture" ("ATS_Async_Ctrl") -> [w351]
          tunnel: w314 -> [w347]
          tunnel: w312 -> [w346]
          tunnel: w299 -> [w341]
          stop <- w345 stop-if-true
          n153 = call "ATS_AsyncDMA_Device.vi"("DeviceIn"=w341, "ATS_Async_Ctrl"=w351) -> ("Buffer"=w349:u16[], "Async_Status"=w344:T38)  [unwired: 9 in, 3 out]
          n154 = local read "Reset DAQ"() -> (w348:bool)
          n155 = call "DAQ Status.vi"("Enum"=DAQ_Status_States."Get", "Async_Status"=w344) -> ("DAQ Error?"=w342:bool, "Valid"=w343:bool)  [unwired: 8 in]
          n156 = Compound Arithmetic op=OR(w342, w348) -> (w345:bool)
          n157 = case shown="True" w343 {
            tunnel: w349 -> [_ w354]
            tunnel: w349 -> [_ w355]
            tunnel: w347 -> [_ w356]
            tunnel: w346 -> [_ w353]
            frame False {
              # "Do nothing"
            }
            frame True {
              w352 = 50 ("timeout in ms (-1)")
              n158 = Enqueue Element(queue=w353, element=w354, timeout in ms (-1)=w352) -> ()  [unwired: 1 in, 3 out]
              n159 = Enqueue Element(queue=w356, element=w355, timeout in ms (-1)=w352) -> ()  [unwired: 1 in, 3 out]
            }
          }
        }
        n160 = while {
          tunnel: [w328] -> w302
          tunnel: w303 -> [w328]
          stop <- w327 stop-if-true
          n161 = local read "Processing Finished"() -> (w327:bool)
          n162 = Wait (ms)(milliseconds to wait=u32 25) -> ()  [unwired: 1 out]
        }
        n163 = call "galvo_functional_global.vi"("State"=galvo_states."Reset", "error in (no error)"=w302) -> ("error out"=w305:errorcluster)  [unwired: 8 in, 1 out]
        n164 = call "Save Data Functional Global.vi"("States"=Saving_Data_States."Close Files", "error in (no error)"=w305) -> ("error out"=w320:errorcluster)  [unwired: 6 in, 3 out]
        n165 = call "Save Data Functional Global.vi"("States"=Saving_Data_States."Do Nothing" ("Save State"), "error in (no error)"=w320) -> ("error out"=w318:errorcluster)  [unwired: 6 in, 3 out]
        n166 = Enqueue Element(queue=w323, element=OCT_Hardware_States."Acquire Data", error in (no error)=w318) -> ()  [unwired: 1 in, 3 out]
      }
      frame "Wait" {
        n167 = Wait (ms)(milliseconds to wait=u32 10) -> ()  [unwired: 1 out]
      }
      frame "Stop" {
        n168 = Release Queue(queue=w368, error in (no error)=w367) -> (error out=w366:errorcluster)  [unwired: 1 in, 2 out]
        n169 = call "OCT Processing 2ch functional global.vi"("State"=processing_states."Shutdown", "error in (no error)"=w366) -> ("error out"=w365:errorcluster)  [unwired: 9 in, 4 out]
        n170 = call "Save Data Functional Global.vi"("States"=Saving_Data_States."Shutdown", "error in (no error)"=w365) -> ("error out"=w362:errorcluster)  [unwired: 6 in, 3 out]
        n171 = call "galvo_functional_global.vi"("State"=galvo_states."Shutdown", "error in (no error)"=w362) -> ("error out"=w361:errorcluster)  [unwired: 8 in, 1 out]
        n172 = flat-sequence {
          tunnel: w361 -> [_]
          frame #0 {
            w372 = 0 ("DeviceIn")
            n173 = call "ATS_AsyncDMA_Device.vi"("DeviceIn"=w372, "ATS_Async_Ctrl"=ATS_Async_Ctrl."Stop") -> ("ReadSamples_Out"=w371:T32)  [unwired: 9 in, 4 out]
            n174 = call "ATS_AsyncDMA_Device.vi"("DeviceIn"=w372, "ATS_Async_Ctrl"=ATS_Async_Ctrl."Abort", "ReadSamples"=w371) -> ()  [unwired: 8 in, 5 out]
          }
          frame #1 {
            n175 = Stop(stop? (T)=TRUE) -> ()
          }
        }
      }
      frame "Initialize Clock" {
        w377 = T16 12 items=["20mV", "40mV", "50mV", "80mV", "100mV", "200mV", "400mV", "500mV", "800mV", "1 V", "1.25 V", "2 V", "4 V", "5 V", "8 V", "10 V", "16 V", "20 V", "40 V", "HiFi"] ("Input B.Range")
        w380 = u32 18 items=["1 kS/s", "2 kS/s", "5 kS/s", "10 kS/s", "20 kS/s", "50 kS/s", "100 kS/s", "200 kS/s", "500 kS/s", "1 MS/s", "2 MS/s", "5 MS/s", "10 MS/s", "20 MS/s", "50 MS/s", "100 MS/s", "125 MS/s", "160 MS/s", "180 MS/s"] ("ClckRate")
        n176 = local read "Clock Length"() -> (w379:u32)
        n177 = call "ATS_Device.vi"("BoardToVerify"=w375, "ATS_Check"=ATS_Check_Ctrl."Verify Board", "DevCtrl"=Device_Ctrl."Initialize", "DeviceIn"=0 ("Device")) -> ("error out"=w382:errorcluster, "DeviceOut"=w387:i32)  [unwired: 1 in, 5 out]
        n178 = Bundle By Name(cluster=w374, "Record.Length"=w379, "Clock.ClckSource"=ClockSource."Internal", "Clock.ClckRate"=w380, "Input B.Range"=w377, "Input A.Impedance"=Impedance."50 ohms") -> (w378:T8)
        n179 = call "ATS_Device.vi"("error in (no error)"=w382, "DevCtrl"=Device_Ctrl."Abort", "DeviceIn"=w387) -> ("DeviceOut"=w385:i32)  [unwired: 2 in, 6 out]
        n180 = call "ATS_MS_Set_Device.vi"("Set_Manually (F)"=FALSE, "Setup_In"=w378, "DeviceIn"=w385) -> ()  [unwired: 3 in, 6 out]
      }
      frame "Set Resampling Array" {
      }
      frame "Update DAQ Parameters" {
        n181 = call "Configure Alazar Cluster.vi"(10:"ATS9462" ("Alazar Board")) -> (3:w392)  [unwired: 10 in]
        n182 = property class="Clust (strict)"(reference=w392) -> ("Value"=w391:T8)  [unwired: 1 in, 2 out]
      }
      frame "K-Space Calibration" {
        n183 = Enqueue Element(queue=w406, element=OCT_Hardware_States."Update DAQ Parameters", error in (no error)=w405) -> (queue out=w394:refnum<queue>, error out=w403:errorcluster)  [unwired: 1 in, 1 out]
        n184 = call "Display Message to User"("error in (no error)"=w403) -> ("error out"=w396:errorcluster)  [unwired: 9 in, 1 out]
        n185 = call "galvo_functional_global.vi"("State"=galvo_states."Center Galvos", "error in (no error)"=w396) -> ("error out"=w395:errorcluster)  [unwired: 8 in, 1 out]
        n186 = Enqueue Element(queue=w394, element=OCT_Hardware_States."Set Resampling Array", error in (no error)=w395) -> (error out=w397:errorcluster)  [unwired: 1 in, 2 out]
        n187 = property on="Calibrate" class="Bool"(error in=w397, "Visible"=TRUE) -> (error out=w399:errorcluster)  [unwired: 1 in, 1 out]
        n188 = property on="Calibrate" class="Bool"(error in=w399, "Blinking"=TRUE) -> ()  [unwired: 1 in, 2 out]
      }
      frame "Background Subtraction" {
        n189 = call "Display Message to User2"("error in (no error)"=w413) -> ("error out"=w414:errorcluster)  [unwired: 9 in, 1 out]
        n190 = call "galvo_functional_global.vi"("State"=galvo_states."Center Galvos", "error in (no error)"=w414) -> ("error out"=w409:errorcluster)  [unwired: 8 in, 1 out]
        n191 = Enqueue Element(queue=w411, element=OCT_Hardware_States."Initialize DAQ", error in (no error)=w409) -> (queue out=w410:refnum<queue>, error out=w408:errorcluster)  [unwired: 1 in, 1 out]
        n192 = Enqueue Element(queue=w410, element=OCT_Hardware_States."Acquire Background", error in (no error)=w408) -> ()  [unwired: 1 in, 3 out]
      }
      frame "Allocate OpenCL Memory" {
      }
      frame "Delete OpenCL Memory" {
      }
    }
  }
  n193 = while {
    tunnel: w11 -> [w420]
    tunnel: w12 -> [w421]
    stop <- FALSE stop-if-true
    # "User Interface Loop"
    n194 = event shown="[4] Menu Selection (User)" {
      selector: w421 -> [_ _ _ _ _ _ _]
      dyn-events: _ -> [_ _ _ _ _ _ _]
      timeout: _ -> [_ _ _ _ _ _ _]
      tunnel: w420 -> [w423 w427 w437 _ w451 _ _]
      event User Event {
        n195 = event-data() -> ("Reset Galvos"=w425:bool)  [unwired: 1 in]
        n196 = local write "Reset DAQ"(w425) -> ()
        n197 = Enqueue Element(queue=w423, element=OCT_Hardware_States."Initialize DAQ") -> ()  [unwired: 2 in, 3 out]
      }
      event "Stop Button": Value Change {
        n198 = event-data() -> ()  [unwired: 1 in, 1 out]
        n199 = flat-sequence {
          tunnel: w427 -> [w431]
          tunnel: [w431] -> w428
          tunnel: [50] -> w426
          tunnel: w428 -> [w433]
          tunnel: w426 -> [w432]
          frame #0 {
            w430 = TRUE ("Reset DAQ")
            n200 = local write "Processing Finished"(w430) -> ()
            n201 = local write "Reset DAQ"(w430) -> ()
          }
          frame #1 {
            n202 = Wait (ms)(milliseconds to wait=w432) -> ()  [unwired: 1 out]
            n203 = Enqueue Element(queue=w433, element=OCT_Hardware_States."Stop") -> ()  [unwired: 2 in, 3 out]
          }
        }
      }
      event "Save Sweep": Value Change {
        n204 = event-data() -> ()  [unwired: 1 in, 1 out]
        n205 = flat-sequence {
          tunnel: [w438] -> w436
          tunnel: w436 -> [w444]
          tunnel: [w442] -> w435
          tunnel: w437 -> [w446]
          tunnel: w435 -> [_]
          frame #0 {
            n206 = call "File Dialog2"("prompt"="Select Path for saving") -> ("selected path"=w438:path)  [unwired: 11 in, 3 out]
          }
          frame #1 {
            n207 = local read "Imaging Parameters"() -> (w441:T4)
            n208 = local write "Save Data"(TRUE ("Save Data")) -> ()
            n209 = call "Save Data Functional Global.vi"("Input Parameters"=w441, "States"=Saving_Data_States."Create Files", "Folder"=w444) -> ("error out"=w442:errorcluster)  [unwired: 5 in, 3 out]
          }
          frame #2 {
            n210 = Enqueue Element(queue=w446, element=OCT_Hardware_States."Aquire and Save") -> ()  [unwired: 2 in, 3 out]
          }
          frame #3 {
            n211 = local write "Reset DAQ"(TRUE ("Reset DAQ")) -> ()
          }
        }
      }
      event User Event {
        n212 = event-data() -> ()  [unwired: 1 in, 1 out]
        n213 = call "OCT Processing 2ch functional global.vi"("State"=processing_states."Get Size") -> ("# elements in queue"=w449:i32)  [unwired: 10 in, 4 out]
        n214 = Equal To 0?(x=w449) -> (x = 0?=→"Processing Finished":bool)
      }
      event Menu Selection (User) {
        n215 = event-data() -> ("ItemTag"=w452:string)  [unwired: 1 in, 2 out]
        n216 = case shown="\"DAQ Status\"" w452 {
          tunnel: w451 -> [_ _ w456 _ _ w468 w472 _]
          frame "Raw Data", Default {
            n217 = call "Display Raw Data.vi"("Enum"=Display_Raw_Data_states."Show") -> ()  [unwired: 11 in]
          }
          frame "DAQ Status" {
            n218 = call "DAQ Status.vi"("Enum"=DAQ_Status_States."Show") -> ()  [unwired: 9 in, 2 out]
          }
          frame "Configure_DAQ" {
            n219 = flat-sequence {
              tunnel: w456 -> [w462]
              tunnel: [w462] -> w455
              frame #0 {
                n220 = local write "Reset DAQ"(TRUE ("Reset DAQ")) -> ()
              }
            }
            n221 = Enqueue Element(queue=w455, element=OCT_Hardware_States."Update DAQ Parameters") -> (queue out=w458:refnum<queue>, error out=w459:errorcluster)  [unwired: 2 in, 1 out]
            n222 = Enqueue Element(queue=w458, element=OCT_Hardware_States."Initialize DAQ", error in (no error)=w459) -> ()  [unwired: 1 in, 3 out]
          }
          frame "En Face" {
            n223 = call "En Face Functional Global.vi"(7:En_Face_States."Show" ("En Face States")) -> ()  [unwired: 9 in, 2 out]
          }
          frame "Save Sweep" {
            n224 = property on="Save Sweep" class="Bool (strict)"("Val(Sgnl)"=TRUE ("Value (Signaling)")) -> ()  [unwired: 2 in, 2 out]
          }
          frame "K-Space Correction" {
            n225 = Enqueue Element(queue=w468, element=OCT_Hardware_States."K-Space Calibration") -> (error out=w466:errorcluster)  [unwired: 2 in, 2 out]
            n226 = flat-sequence {
              tunnel: w466 -> [_]
              tunnel: [TRUE] -> w465
              frame #0 {
              }
            }
            n227 = local write "Reset DAQ"(w465) -> ()
          }
          frame "Background Subtraction" {
            n228 = Enqueue Element(queue=w472, element=OCT_Hardware_States."Background Subtraction") -> (error out=w471:errorcluster)  [unwired: 2 in, 2 out]
            n229 = flat-sequence {
              tunnel: [w475] -> _
              tunnel: w471 -> [w475]
              tunnel: [TRUE ("Reset DAQ")] -> w470
              frame #0 {
              }
            }
            n230 = local write "Reset DAQ"(w470) -> ()
          }
          frame "Configure_Galvos" {
            n231 = call "galvo_functional_global.vi"("State"=galvo_states."Show") -> ()  [unwired: 9 in, 2 out]
          }
        }
      }
      event "Save Sweep Button": Value Change {
        n232 = event-data() -> ()  [unwired: 1 in, 1 out]
        n233 = property on="Save Sweep" class="Bool (strict)"("Val(Sgnl)"=TRUE ("Value (Signaling)")) -> ()  [unwired: 2 in, 2 out]
      }
      event "Calibrate": Value Change {
        n234 = event-data() -> ()  [unwired: 1 in, 1 out]
        n235 = property on="Calibrate" class="Bool"("Visible"=FALSE) -> (error out=w482:errorcluster)  [unwired: 2 in, 1 out]
        n236 = property on="Calibrate" class="Bool"(error in=w482, "Blinking"=FALSE) -> ()  [unwired: 1 in, 2 out]
        n237 = call "Display Raw Data.vi"("Enum"=Display_Raw_Data_states."Add Raw") -> ()  [unwired: 11 in]
        n238 = call "Clock Frequency generator hilbert without wavepond.vi"() -> ("Zero Crossing Resample Index"=w478:i32[])  [unwired: 11 in]
        n239 = call "OCT Processing 2ch functional global.vi"("State"=processing_states."Set Reample Array", "Resample Array"=w478) -> ()  [unwired: 9 in, 5 out]
      }
    }
  }
  n240 = while {
    stop <- w491 stop-if-true
    # "Display Loop"
    # "Sometimes a timeout event sends\na 0 array, this stops the flickering\nof the front panl due to those \ntimeout events"
    # "This takes the 0th element of the processed data,\nthe other elements will NOT be displayed"
    # "This loop just gets the last b-scan processed wheter in real time mode or not. \nJust meant to update the front panel Asynchronously.  This frame is NOT\nguarenteed to view every BScan, just the last one processed."
    n241 = call "OCT Processing 2ch functional global.vi"("State"=processing_states."Get Last Processed BScan") -> ("Processed OCT Data"=w488:T30)  [unwired: 10 in, 4 out]
    n242 = case shown="\"Channel A\", Default" "Display" {
      tunnel: w488 -> [w496 w497]
      tunnel: [w494 w498] -> w486
      frame "Channel A", Default {
        n243 = Unbundle By Name(w496) -> ("Intensity A"=w495:sgl[][][])
        n244 = Index Array(array=w495) -> (element=w494:sgl[][])  [unwired: 3 in]
      }
      frame "Channel B" {
        n245 = Unbundle By Name(w497) -> ("Intensity B"=w499:sgl[][][])
        n246 = Index Array(array=w499) -> (element=w498:sgl[][])  [unwired: 3 in]
      }
    }
    n247 = Array Size(array=w486) -> (size(s)=w487:i32[])
    n248 = Multiply Array Elements(1:w487) -> (0:w485:i32)
    n249 = Equal To 0?(x=w485) -> (x = 0?=w484:bool)
    n250 = case shown="False" w484 {
      tunnel: w486 -> [w492 _]
      frame False {
        "BScan" <- w492
      }
      frame True {
        n251 = Wait Until Next ms Multiple(millisecond multiple=u32 10) -> ()  [unwired: 1 out]
      }
    }
    n252 = local read "Stop Button"() -> (w491:bool)
  }
